vi "Fpga-OrderBook-TestHarness.vi"   [LabVIEW 2016]
uses:
  <vilib>/Platform/TimedLoop/XDataNode/timing_clust.ctl
  <vilib>/Platform/TimedLoop/XDataNode/nitl_modes.ctl
  <vilib>/Platform/TimedLoop/XDataNode/wakeup.ctl
  <vilib>/rvi/Emulation/niFpgaSctlEmulationGetInTimedLoop.vi
  <vilib>/rvi/Emulation/niFpgaEmulationReportErrorSimple.vi
  <vilib>/rvi/Emulation/niFpgaGetClockAttributes.vi
  <vilib>/rvi/Emulation/niFpgaCriticalErrorInLSC.vi
  <vilib>/rvi/interface/RandomDataEmulation/niFpgaRandomDataHandleErrors.vi
  <vilib>/rvi/Emulation/niFpgaEmulationIsFPGAContextNoSignature.vi
  <vilib>/rvi/errors/niFpgaSetErrorForExecOnDevCompSimple.vi
  <vilib>/rvi/eio/common/nirviEmuReportErrorAndStop.vi
  <vilib>/rvi/DataTransferAndStorage/Container/Common/niFpgaContainerGetUniqueNameForEmu.vi
  <vilib>/rvi/FIFO/Fifo_Resource/nirvififoEmulationSetSize.vi
  <vilib>/rvi/FIFO/Fifo_Resource/nirviFifoEmulationQueueMgr.vi
  <instcachedir>/0/nirviFifoEmulationQueueMgr_E5CAEC123FF24DC58D834DCA3CDAA9B5.lvgen/nirviFifoEmulationQueueMgr_E5CAEC123FF24DC58D834DCA3CDAA9B5_010.vi
  <vilib>/rvi/FIFO/Fifo_Resource/nirvififoEmulationDetermineInputValidOut.vi
  <vilib>/rvi/FIFO/Fifo_Resource/nirvififoEmulationCreateLock.vi
  <vilib>/rvi/Emulation/niFpgaProcessEmulError.vi
  <vilib>/rvi/FIFO/Fifo_Resource/nirvififoEmulationObtainLock.vi
  <vilib>/rvi/FIFO/Fifo_Resource/nirvififoEmulationReleaseLock.vi
  <vilib>/rvi/occurrence/nirviWaitOnOccurrenceBase.vi
  <vilib>/rvi/errors/nirviReportUnexpectedCaseInternalError.vi
  <vilib>/rvi/errors/nirviReportUnexpectedCaseInternalError (U32).vi
  <instcachedir>/0/nirviFifoEmulationQueueMgr_E5CAEC123FF24DC58D834DCA3CDAA9B5.lvgen/nirviFifoEmulationQueueMgr_E5CAEC123FF24DC58D834DCA3CDAA9B5_011.vi
  <vilib>/Utility/error.llb/Clear Errors.vi
  <vilib>/Platform/TimedLoop/XDataNode/XDataNode.xnode
  <vilib>/rvi/DataTransferAndStorage/Container/XNode/niFpgaContainer.xnode
  <vilib>/rvi/interface/RandomDataEmulation/nirviRandomDataFpgaReadWriteTemplate.vi
  <vilib>/rvi/FIFO/Fifo_Resource/nirvififoEmulationWrite.vi
  <vilib>/rvi/FIFO/Fifo_Resource/nirvififoEmulationRead.vi
  <vilib>/Platform/TimedLoop/XDataNode/XDNodeRunTimeDep.lvlib
types:
  T1 = cluster{"Side":enum16{"Sell", "Buy"}, "OrderRefNum":u64, "Price":u32, "Shares":u32}
  T2 = cluster{"Operation":enum16{"Noop", "GetAll", "AddOrder", "DeleteOrder"}, "Cluster":cluster{"Side":enum16{"Sell", "Buy"}, "OrderRefNum":u64, "Price":u32, "Shares":u32}}
  T3 = typedef "XDNodeRunTimeDep.lvlib/timing_clust.ctl" = cluster{"Expected End [f-1]":u64, "Actual End [f-1]":u64, "Finished Late? [f-1]":bool, "Expected End [i-1]":u64, "Actual End [i-1]":u64, "Finished Late? [i-1]":bool, "Expected Start [i]":u64, "Actual Start [i]":u64, "Expected Start [f]":u64, "Actual Start [f]":u64, "Source Name":string, "Structure Name":string, "Period":i64, "Deadline":i64, "Offset":i64, "Start":i64, "Priority":i32, "Timeout":i32, "Mode":T4, "Wakeup Reason":T5, "Error":errorcluster, "Source Type":string, "Secondary Source Type":string, "Global End Time":u64, "Global Start Time":u64, "Frame Duration":u64, "Iteration Duration":u64, "Assigned CPU":i32, "I/O Scan Engine Mode":u32}
  T4 = typedef "XDNodeRunTimeDep.lvlib/nitl_modes.ctl" = enum32{"No Change", "Process missed periods, maintain original phase", "Discard missed periods, maintain original phase", "Process missed periods, ignore original phase", "Discard missed periods, ignore original phase"}
  T5 = typedef "XDNodeRunTimeDep.lvlib/wakeup.ctl" = enum32{"Normal", "Aborted", "Asynchronous wakeup", "Timing source error", "Timed loop error", "Timeout"}
  T6 = enum16{"Noop", "GetAll", "AddOrder", "DeleteOrder"}
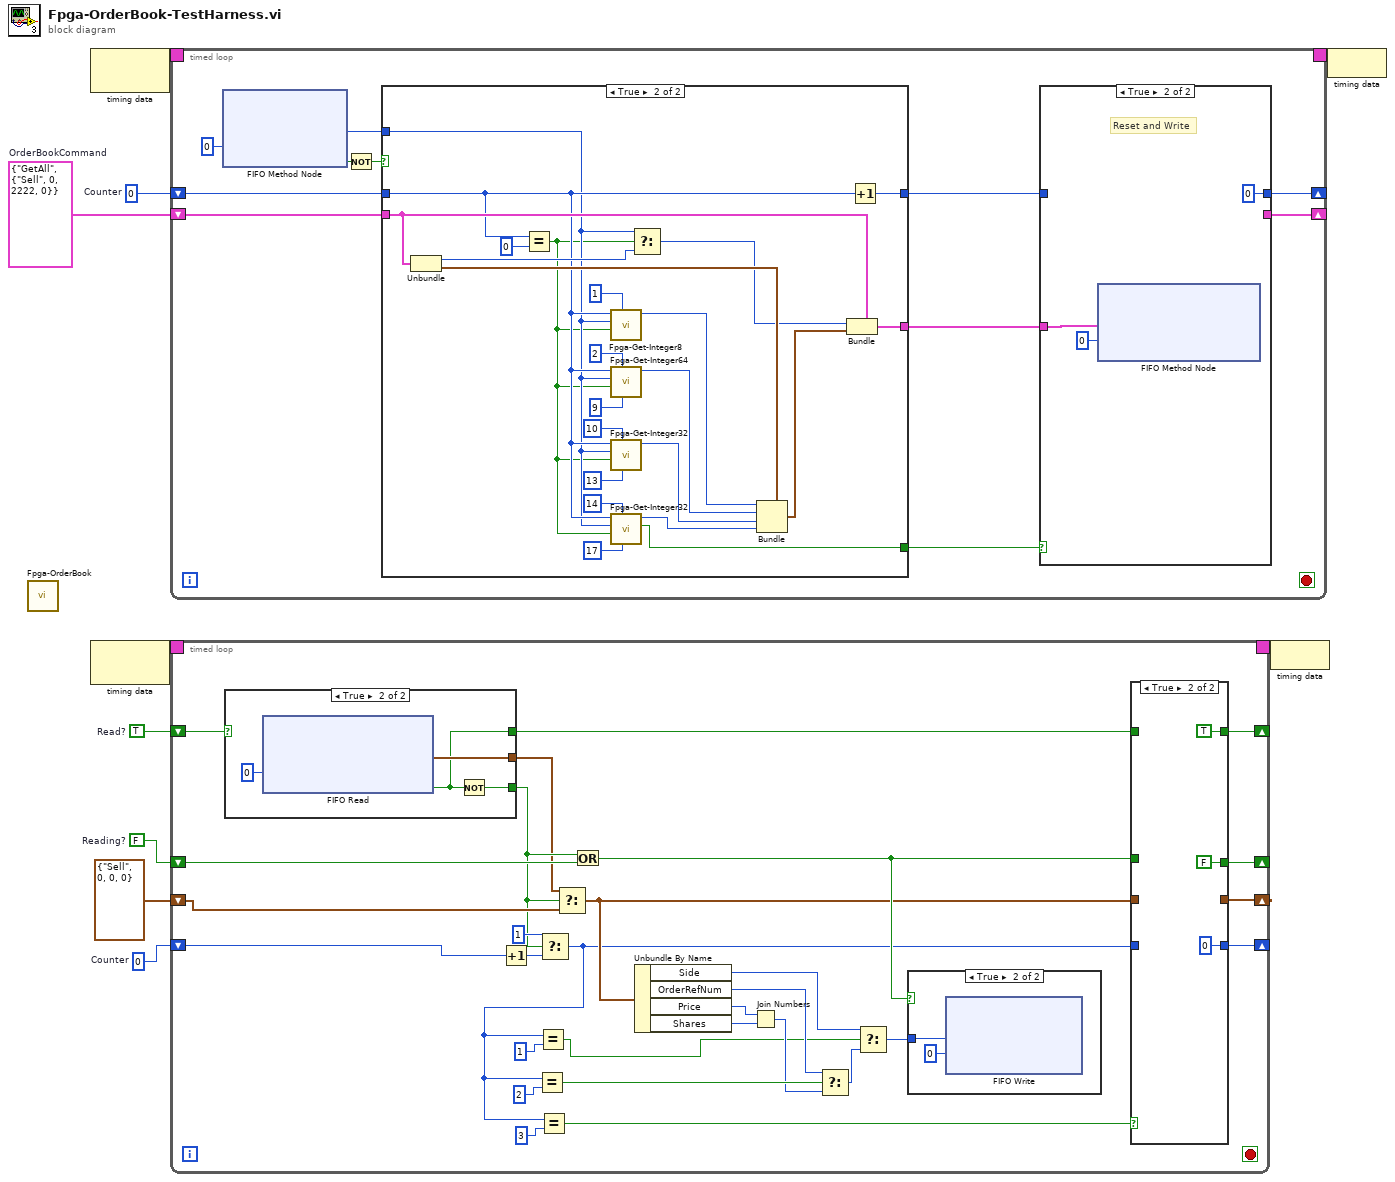
[diagram p0: block diagram]
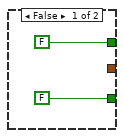
[diagram p4: hidden frame]
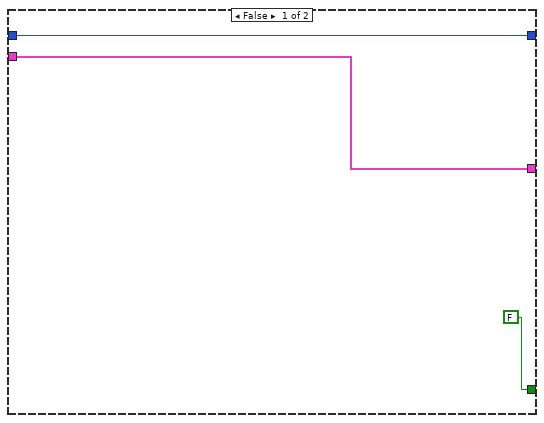
[diagram p6: hidden frame]
diagram:
  w2 = u16 0  # Counter
  w3 = T2 {"Operation"=enum."GetAll", "Cluster"={"Side"=enum."Sell", "OrderRefNum"=0, "Price"=2222, "Shares"=0}}  # OrderBookCommand
  w4 = FALSE  # Reading?
  w5 = i16 0  # Counter
  w6 = TRUE  # Read?
  n1 = call "Fpga-OrderBook.vi"() -> ()  [unwired: 12 in]
  n2 = node-c288() -> (w10:T3)  [unwired: 1 in]
  n3 = node-c288() -> (w8:T3)  [unwired: 1 in]
  n4 = timed-loop {
    timing: w10 -> [_]
    timing-out: [_] -> w9
    shift-right: [w14] -> _
    shift-left: w3 -> [w17]
    shift-right: [w15] -> _
    shift-left: w2 -> [w18]
    stop <- _ stop-if-true
    n5 = xnode ("FIFO Method Node")("Timeout"=0) -> ("Element"=w16:u8, "Timed Out?"=w20:bool)  [unwired: 1 in, 1 out]
    n6 = Not(x=w20) -> (.not. x?=w19:bool)
    n7 = case shown="True" w19 {
      tunnel: w18 -> [w28 w34]
      tunnel: [w28 w52] -> w12
      tunnel: w17 -> [w29 w50]
      tunnel: w16 -> [_ w32]
      tunnel: [w29 w47] -> w11
      tunnel: [FALSE w43] -> w13
      frame False {
      }
      frame True {
        n8 = Unbundle(w50) -> ("Operation"=w48:T6, "Cluster"=w46:T1)
        n9 = Equal?(x=w34, y=u16 0) -> (x = y?=w31:bool)
        n10 = call "Fpga-Get-Integer8.vi"("lower"=u16 1, "Reset"=w31, "DataIn"=w32, "Index"=w34) -> ("U8"=w30:u8)  [unwired: 6 in, 1 out]
        n11 = call "Fpga-Get-Integer64.vi"("upper"=u16 9, "lower"=u16 2, "Reset"=w31, "DataIn"=w32, "Index"=w34) -> ("UInt32"=w42:u64)  [unwired: 5 in, 1 out]
        n12 = call "Fpga-Get-Integer32.vi"("upper"=u16 13, "lower"=u16 10, "Reset"=w31, "DataIn"=w32, "Index"=w34) -> ("UInt32"=w44:u32)  [unwired: 5 in, 1 out]
        n13 = call "Fpga-Get-Integer32.vi"("upper"=u16 17, "lower"=u16 14, "Reset"=w31, "DataIn"=w32, "Index"=w34) -> ("Valid"=w43:bool, "UInt32"=w45:u32)  [unwired: 5 in]
        n14 = Select(t=w32, s=w31, f=w48) -> (s? t:f=w41:u16)
        n15 = Bundle(cluster=w46, "Side"=w30, "OrderRefNum"=w42, "Price"=w44, "Shares"=w45) -> (w49:T1)
        n16 = Bundle(cluster=w50, "Operation"=w41, "Cluster"=w49) -> (w47:T2)
        n17 = Increment(x=w34) -> (x+1=w52:u16)
      }
    }
    n18 = case shown="True" w13 {
      tunnel: w12 -> [w23 _]
      tunnel: w11 -> [w22 w24]
      tunnel: [w23 u16 0 ("Counter")] -> w15
      tunnel: [w22 _] -> w14
      frame False {
      }
      frame True {
        # "Reset and Write"
        n19 = xnode ("FIFO Method Node")("Element"=w24, "Timeout"=0) -> ()  [unwired: 1 in, 2 out]
      }
    }
  }
  n20 = timed-loop {
    timing: w8 -> [_]
    timing-out: [_] -> w7
    shift-right: [w81] -> _
    shift-left: w6 -> [w82]
    shift-right: [w79] -> _
    shift-left: w5 -> [w57]
    shift-right: [w77] -> _
    shift-left: w4 -> [w78]
    shift-right: [w74] -> _
    shift-left: T1 {"Side"=enum."Sell", "OrderRefNum"=0, "Price"=0, "Shares"=0} ("Cluster") -> [w73]
    stop <- _ stop-if-true
    n21 = case shown="True" w82 {
      tunnel: [_ w97] -> w60
      tunnel: [FALSE ("Timed Out?") w96] -> w61
      tunnel: [FALSE w95] -> w80
      frame False {
      }
      frame True {
        n22 = xnode ("FIFO Read")("Timeout"=0) -> ("Element"=w97:T1, "Timed Out?"=w95:bool)  [unwired: 1 in, 1 out]
        n23 = Not(x=w95) -> (.not. x?=w96:bool)
      }
    }
    n24 = Increment(x=w57) -> (x+1=w83:i16)
    n25 = Select(t=i16 1, s=w61, f=w83) -> (s? t:f=w56:i16)
    n26 = Equal?(x=w56, y=i16 2) -> (x = y?=w68:bool)
    n27 = Equal?(x=w56, y=i16 1) -> (x = y?=w58:bool)
    n28 = Equal?(x=w56, y=i16 3) -> (x = y?=w63:bool)
    n29 = Select(t=w60, s=w61, f=w73) -> (s? t:f=w62:T1)
    n30 = Or(x=w61, y=w78) -> (x .or. y?=w75:bool)
    n31 = Unbundle By Name(w62) -> ("Side"=w59:enum16{"Sell", "Buy"}, "OrderRefNum"=w67:u64, "Price"=w66:u32, "Shares"=w65:u32)
    n32 = Join Numbers(hi=w66, lo=w65) -> ((hi.lo)=w64:u64)
    n33 = Select(t=w67, s=w68, f=w64) -> (s? t:f=w69:u64)
    n34 = Select(t=w59, s=w58, f=w69) -> (s? t:f=w55:u64)
    n35 = case shown="True" w75 {
      tunnel: w55 -> [_ w84]
      frame False {
      }
      frame True {
        n36 = xnode ("FIFO Write")("Element"=w84, "Timeout"=0) -> ()  [unwired: 1 in, 2 out]
      }
    }
    n37 = case shown="True" w63 {
      tunnel: [w89 TRUE ("Timed Out?")] -> w81
      tunnel: w80 -> [w89 _]
      tunnel: w56 -> [w88 _]
      tunnel: [w88 i16 0 ("Counter")] -> w79
      tunnel: w75 -> [w87 _]
      tunnel: [w87 FALSE] -> w77
      tunnel: [w86 _] -> w74
      tunnel: w62 -> [w86 _]
      frame False {
      }
      frame True {
      }
    }
  }
  n38 = node-c288(w7) -> ()
  n39 = node-c288(w9) -> ()
